vi "GetChiChoice.vi"(9 "Tile":u16(ring), 10 "Hand":u16[](array[ring])) -> (2 "ChiChoice":u16[][](array[ring]))   [LabVIEW 2025]
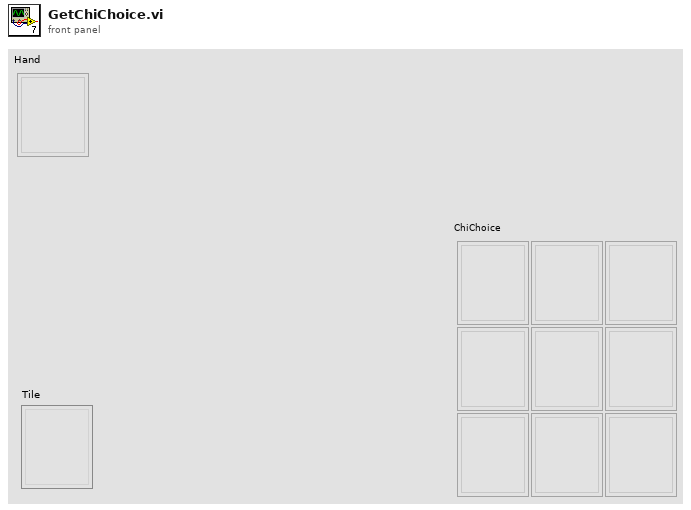
[diagram p1: front panel]
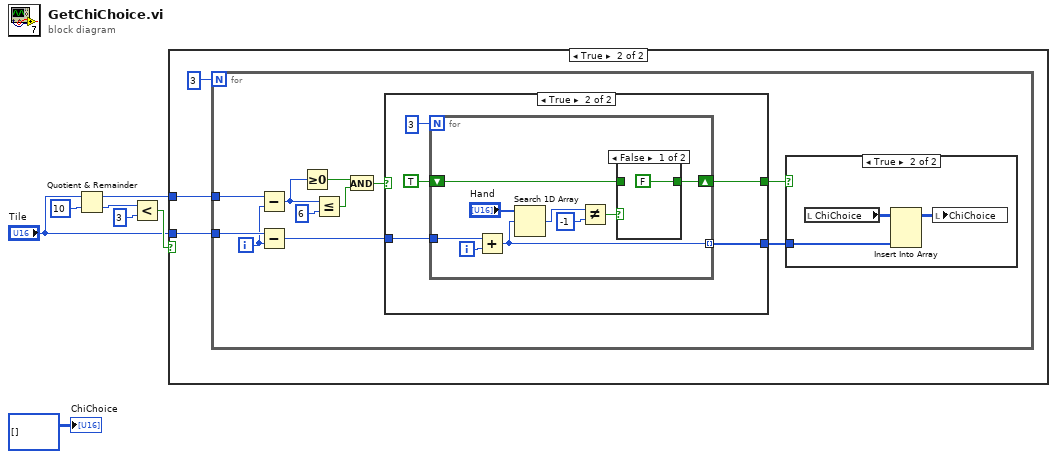
[diagram p0: block diagram]
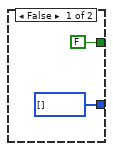
[diagram p4: hidden frame]
diagram:
  n1 = Quotient & Remainder(x="Tile", y=10) -> (x-y*floor(x/y)=w3:i32, floor(x/y)=w6:i32)
  n2 = Less?(x=w6, y=3) -> (x < y?=w4:bool)
  n3 = case shown="True" w4 {
    tunnel: w3 -> [_ w9]
    tunnel: "Tile" -> [_ w8]
    frame False {
    }
    frame True {
      n4 = for {
        N: 3 -> [_]
        tunnel: w9 -> [w21]
        tunnel: w8 -> [w15]
        i -> [w14]
        n5 = Subtract(x=w21, y=w14) -> (x-y=w19:i32)
        n6 = Subtract(x=w15, y=w14) -> (x-y=w13:i32)
        n7 = Greater Or Equal To 0?(x=w19) -> (x >= 0?=w16:bool)
        n8 = Less Or Equal?(x=w19, y=6) -> (x <= y?=w17:bool)
        n9 = And(x=w16, y=w17) -> (x .and. y?=w18:bool)
        n10 = case shown="True" w18 {
          tunnel: w13 -> [_ w30]
          tunnel: [FALSE w29] -> w12
          tunnel: [i32[] [] w27] -> w11
          frame False {
          }
          frame True {
            n11 = for {
              N: 3 -> [_]
              tunnel: w30 -> [w40]
              tunnel: [w35] -> w27 mode=indexing
              shift-right: [w33] -> w29
              shift-left: TRUE -> [w34]
              i -> [w39]
              n12 = Add(x=w40, y=w39) -> (x+y=w35:i32)
              n13 = Search 1D Array(1D array="Hand", element=w35) -> (index of element=w37:i32)  [unwired: 1 in]
              n14 = Not Equal?(x=w37, y=-1) -> (x != y?=w38:bool)
              n15 = case shown="False" w38 {
                tunnel: w34 -> [_ w42]
                tunnel: [FALSE w42] -> w33
                frame False {
                }
                frame True {
                }
              }
            }
          }
        }
        n16 = case shown="True" w12 {
          tunnel: w11 -> [_ w23]
          frame False {
          }
          frame True {
            n17 = local read "ChiChoice"() -> (w24:u16[][])
            n18 = Insert Into Array(array=w24, new element=w23) -> (w22:u16[][])  [unwired: 2 in]
            n19 = local write "ChiChoice"(w22) -> ()
          }
        }
      }
    }
  }
  "ChiChoice" <- i32[][] []
